vi "LJM logger conditionally clear input errors.vi"(1 "error in":errorcluster) -> (0 "error out":errorcluster)   [LabVIEW 2026]
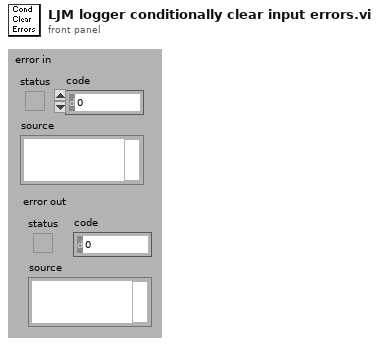
[diagram p1: front panel]
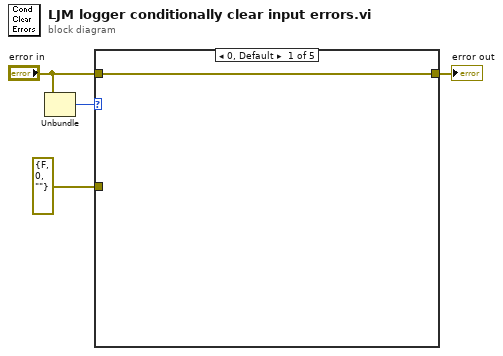
[diagram p0: block diagram]
diagram:
  n1 = Unbundle("error in") -> ("code"=w4:i32)  [unwired: 2 out]
  n2 = case shown="0, Default" w4 {
    tunnel: "error in" -> [w5 _ _ _ _]
    tunnel: [w5 w6 w7 w8 w9] -> w2
    tunnel: errorcluster {"status"=FALSE, "code"=0, "source"=""} ("error in") -> [_ w6 w7 w8 w9]
    frame 0, Default {
    }
    frame 7294 {
      # "If the error is LJME_INVALID_NAME, clear the error"
    }
    frame 7239 {
      # "Ignore reconnection errrors"
    }
    frame 2583 {
      # "If the error is AIN_EF_CHANNEL_INACTIVE, clear the error"
    }
    frame 2377 {
      # "If the error is AIN_CHN_DISABLED, clear the error"
    }
  }
  "error out" <- w2
